vi "Main.vi"() -> ()   [LabVIEW 2023]
panel:
  in  "Save":bool
  in  "stop":bool
  in  "Phone Number":string
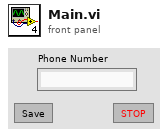
[diagram p1: front panel]
types:
  T1 = enum16{"open", "replace", "create", "open or create", "replace or create", "replace or create with confirmation"}
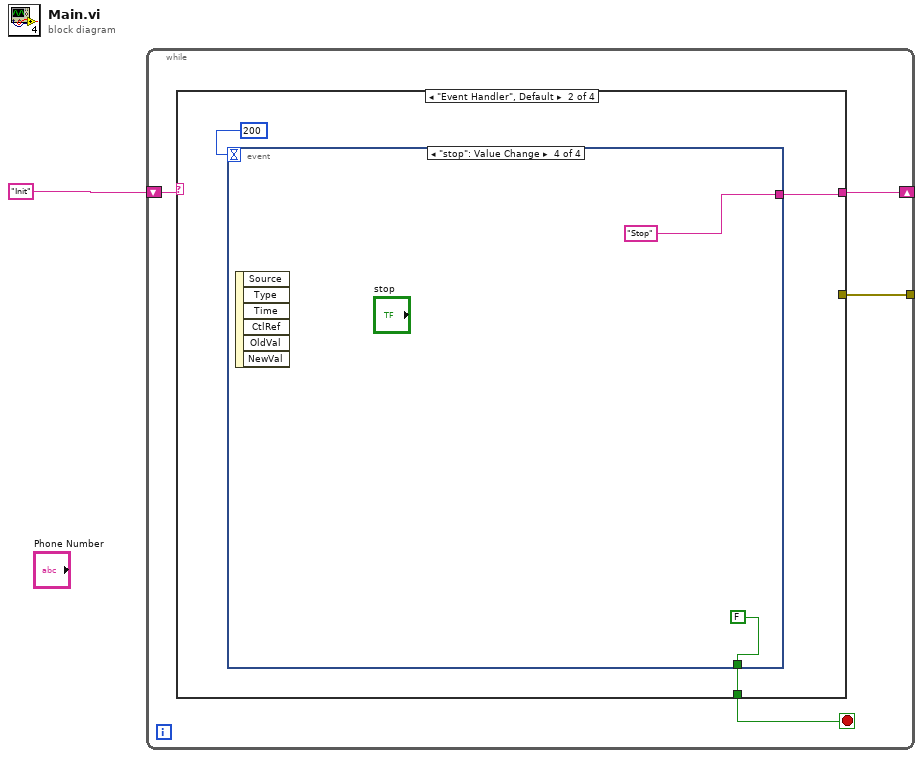
[diagram p0: block diagram]
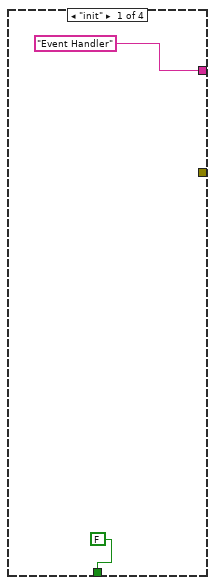
[diagram p2: hidden frame]
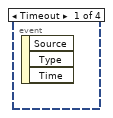
[diagram p3: hidden frame]
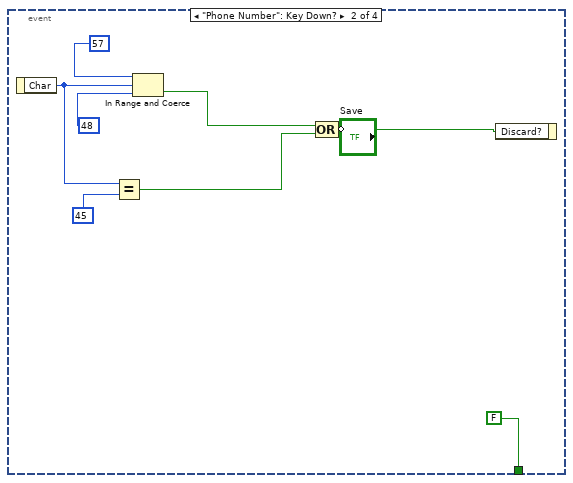
[diagram p4: hidden frame]
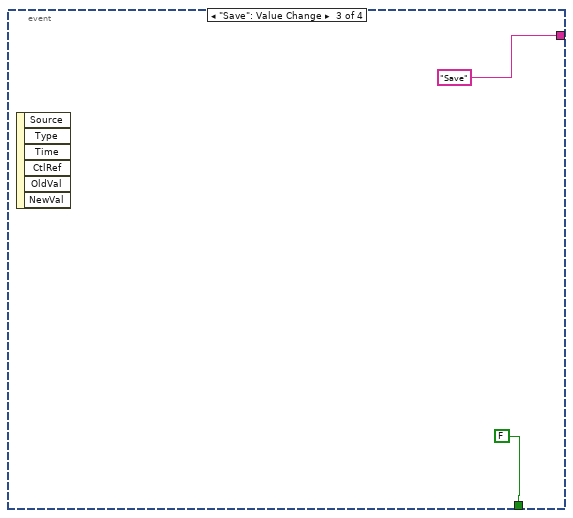
[diagram p5: hidden frame]
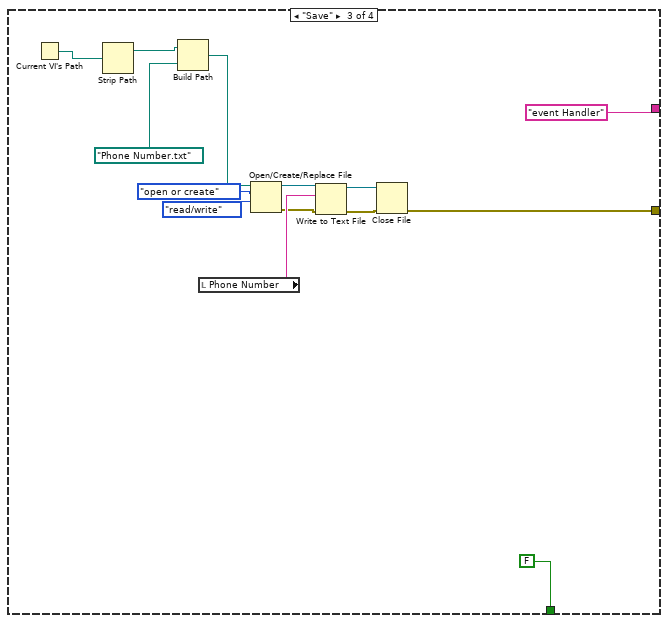
[diagram p6: hidden frame]
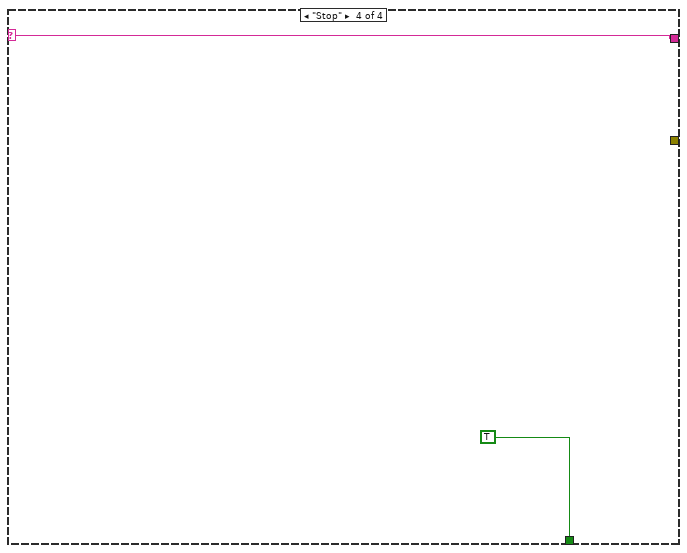
[diagram p7: hidden frame]
diagram:
  n1 = while {
    shift-right: [w3] -> _
    shift-left: "Init" -> [w4]
    tunnel: [w2] -> _
    stop <- w5 stop-if-true
    n2 = case shown="\"Event Handler\", Default" w4 {
      selector: w4 -> [_ _ _ w37]
      tunnel: [FALSE w10 FALSE TRUE] -> w5
      tunnel: ["Event Handler" w9 "event Handler" w37] -> w3
      tunnel: [_ _ w23 _] -> w2
      frame "init" {
      }
      frame "Event Handler", Default {
        n3 = event shown="[3] \"stop\": Value Change" {
          selector: _ -> [_ _ _ _]
          dyn-events: _ -> [_ _ _ _]
          timeout: 200 -> [_ _ _ _]
          tunnel: [_ FALSE FALSE FALSE] -> w10
          tunnel: [_ _ "Save" "Stop"] -> w9
          event Timeout {
            n4 = event-data() -> ()  [unwired: 1 in, 3 out]
          }
          event "Phone Number": Key Down? {
            n5 = event-data() -> ("Char"=w16:i16)  [unwired: 1 in]
            n6 = Equal?(x=w16, y=i16 45) -> (x = y?=w13:bool)
            n7 = In Range and Coerce(upper limit=i16 57, x=w16, lower limit=i16 48) -> (In Range?=w14:bool)  [unwired: 1 out]
            n8 = Compound Arithmetic op=OR(w14, w13) -> (invert w12:bool)
            n9 = event-data("Discard?"=w12) -> ()  [unwired: 1 in, 1 out]
          }
          event "Save": Value Change {
            n10 = event-data() -> ()  [unwired: 1 in, 6 out]
          }
          event "stop": Value Change {
            n11 = event-data() -> ()  [unwired: 1 in, 6 out]
          }
        }
      }
      frame "Save" {
        n12 = Current VI's Path() -> (path=w34:path)
        n13 = Strip Path(path=w34) -> (stripped path=w33:path)  [unwired: 1 out]
        n14 = Build Path(base path=w33, name or relative path=path "Phone Number.txt") -> (appended path=w31:path)
        n15 = local read "Phone Number"() -> (w27:string)
        n16 = Open/Create/Replace File(file path (use dialog)=w31, operation (0:open)=T1."open or create", access (0:read/write)=enum16{"read/write", "read-only", "write-only"}."read/write") -> (refnum out=w28:refnum<file>, error out=w26:errorcluster)  [unwired: 3 in, 1 out]
        n17 = Write to Text File(file (use dialog)=w28, text=w27, error in=w26) -> (refnum out=w25:refnum<file>, error out=w24:errorcluster)  [unwired: 1 in, 1 out]
        n18 = Close File(refnum=w25, error in=w24) -> (error out=w23:errorcluster)  [unwired: 1 out]
      }
      frame "Stop" {
      }
    }
  }
